vi "Update Sensor Number.vi"(8 "error in (no error)":errorcluster, 10 "Event Data":i32, 11 "Main View in":refnum<class "Main View.lvclass">) -> (0 "error out":errorcluster, 3 "Main View out":refnum<class "Main View.lvclass">)   [LabVIEW 2013, in "Main View.lvlib" / "Main View.lvclass"]
uses:
  Main View.lvclass
  Main View.lvclass/Main View.ctl
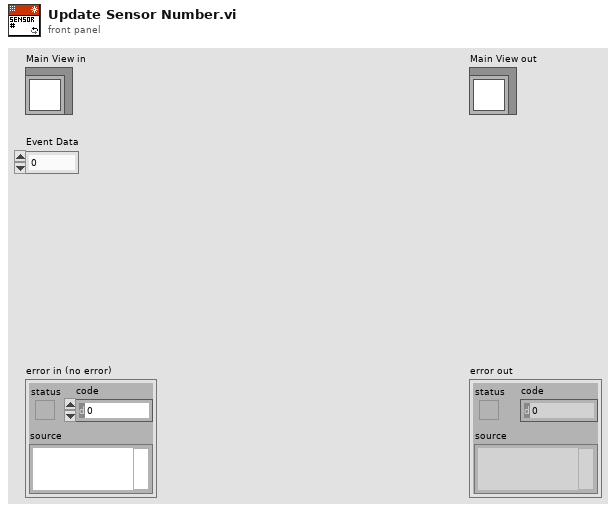
[diagram p1: front panel]
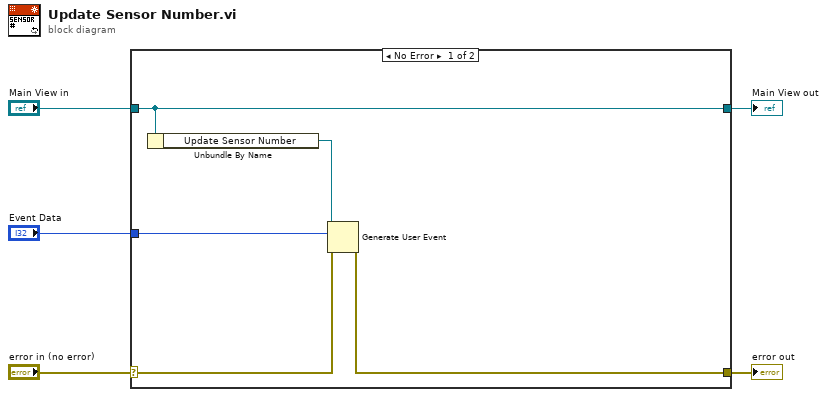
[diagram p0: block diagram]
diagram:
  n1 = case shown="No Error" "error in (no error)" {
    selector: "error in (no error)" -> [w7 w12]
    tunnel: [w6 w12] -> w4
    tunnel: [w10 w11] -> w2
    tunnel: "Main View in" -> [w10 w11]
    tunnel: "Event Data" -> [w8 _]
    frame No Error {
      n2 = Unbundle By Name(w10) -> ("Update Sensor Number"=w9:refnum<user-event>)
      n3 = Generate User Event(user event=w9, event data cluster=w8, error in=w7) -> (error out=w6:errorcluster)  [unwired: 1 in, 1 out]
    }
    frame Error {
    }
  }
  "error out" <- w4
  "Main View out" <- w2
